vi "Parse String.vi"(9 "Start Index":i32, 10 "JSON":string) -> (1 "String":string, 2 "EndIndex":i32, 3 "JSON":string)   [LabVIEW 2011]
panel:
  out "StartIndex":i32
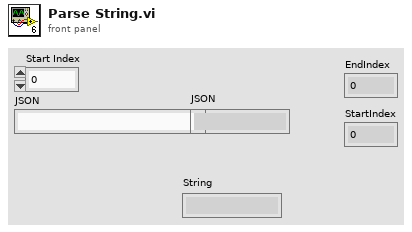
[diagram p1: front panel]
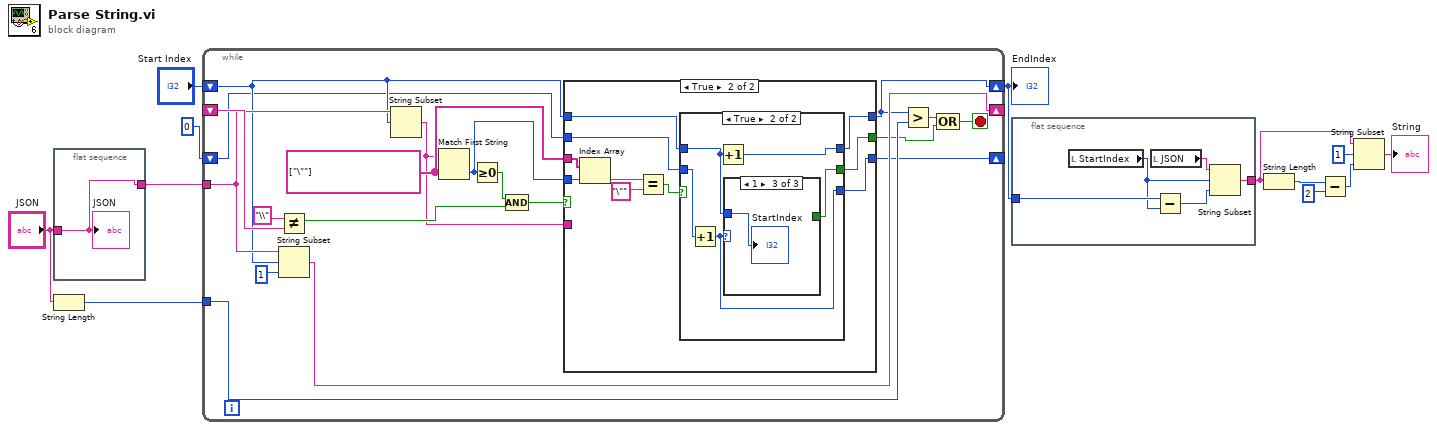
[diagram p0: block diagram]
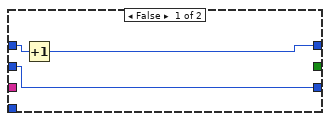
[diagram p2: hidden frame]
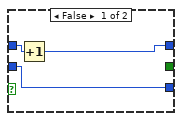
[diagram p3: hidden frame]
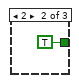
[diagram p5: hidden frame]
diagram:
  n1 = flat-sequence {
    tunnel: "JSON" -> [w13]
    tunnel: [w13] -> w7
    frame #0 {
      "JSON" <- w13
    }
  }
  n2 = String Length(string="JSON") -> (length=w11:i32)
  n3 = while {
    tunnel: w7 -> [w27]
    shift-right: [w20] -> w9
    shift-left: "Start Index" -> [w21]
    tunnel: w11 -> [w32]
    shift-right: [w31] -> _
    shift-left: _ -> [w29]
    shift-right: [w14] -> _
    shift-left: 0 -> [w18]
    stop <- w16 stop-if-true
    w23 = string[] ["\""] ("string array")
    n4 = Not Equal?(x="\\", y=w29) -> (x != y?=w25:bool)
    n5 = String Subset(string=w27, offset (0)=w21, length (rest)=1 ("length (rest)")) -> (substring=w31:string)
    n6 = String Subset(string=w27, offset (0)=w21) -> (substring=w19:string)  [unwired: 1 in]
    n7 = Match First String(2:w23, 3:w19) -> (0:w22:i32)  [unwired: 1 out]
    n8 = Greater Or Equal To 0?(x=w22) -> (x >= 0?=w26:bool)
    n9 = Compound Arithmetic op=AND(w26, w25) -> (w24:bool)
    n10 = case shown="True" w24 {
      tunnel: w23 -> [_ w45]
      tunnel: w22 -> [_ w44]
      tunnel: w21 -> [w35 w39]
      tunnel: [w34 w40] -> w20
      tunnel: w19 -> [_ _]
      tunnel: w18 -> [w33 w38]
      tunnel: [_ w37] -> w15
      tunnel: [w33 w36] -> w14
      frame False {
        n11 = Increment(x=w35) -> (x+1=w34:i32)
      }
      frame True {
        n12 = Index Array(array=w45, index=w44) -> (element=w43:string)
        n13 = Equal?(x=w43, y="\"") -> (x = y?=w41:bool)
        n14 = case shown="True" w41 {
          tunnel: [w47 w52] -> w40
          tunnel: w39 -> [w48 w50]
          tunnel: w38 -> [w46 w53]
          tunnel: [_ w49] -> w37
          tunnel: [w46 w51] -> w36
          frame False {
            n15 = Increment(x=w48) -> (x+1=w47:i32)
          }
          frame True {
            n16 = Increment(x=w53) -> (x+1=w51:i32)
            n17 = Increment(x=w50) -> (x+1=w52:i32)
            n18 = case shown="1" w51 {
              tunnel: w50 -> [_ _ w55]
              tunnel: [_ TRUE _] -> w49
              frame Default {
              }
              frame 2 {
              }
              frame 1 {
                "StartIndex" <- w55
              }
            }
          }
        }
      }
    }
    n19 = Greater?(x=w20, y=w32) -> (0:w17:bool)
    n20 = Compound Arithmetic op=OR(w17, w15) -> (w16:bool)
  }
  "EndIndex" <- w9
  n21 = flat-sequence {
    tunnel: w9 -> [w59]
    tunnel: [w56] -> w5
    frame #0 {
      n22 = local read "StartIndex"() -> (w58:i32)
      n23 = local read "JSON"() -> (w60:string)
      n24 = Subtract(x=w59, y=w58) -> (x-y=w57:i32)
      n25 = String Subset(string=w60, offset (0)=w58, length (rest)=w57) -> (substring=w56:string)
    }
  }
  n26 = String Length(string=w5) -> (length=w3:i32)
  n27 = Subtract(x=w3, y=2) -> (x-y=w1:i32)
  n28 = String Subset(string=w5, offset (0)=1, length (rest)=w1) -> (substring=→"String":string)
